vi "pmu_Read CFG3.vi"(8 "error in (no error)":errorcluster, 11 "system info in":refnum<class "PMU System Info.lvclass">) -> (0 "error out":errorcluster, 2 "CFG-3":T1={"station name"="", "PMU ID"=0, "global PMU ID"=10000000, "time base"=1, "nominal frequency"=enum."60 Hz", "reporting rate"=0, "phasor number"=0, "analog number"=0, "digital number"=0, "channel names"=[], "phasor scale first 4 bytes"=[], "phasor scale factors"=[], "phasor angle offsets [rad]"=[], "analog scale factors"=[], "analog magnitude offsets"=[], "digital units"=[], "data format"=15, "number of PMUs"=1} {"digital units" format="%.0x"}, 3 "system info out":refnum<class "PMU System Info.lvclass">)   [LabVIEW 2013, in "NI_EP_PMU.lvlib" / "PMU System Info.lvclass"]
uses:
  <vilib>/addons/Electrical Power/PMU/Common/Classes/PMU System Info/PMU System Info.lvclass
  <vilib>/addons/Electrical Power/PMU/Common/Controls/pmu_CFG-3 Class.ctl
  <vilib>/addons/Electrical Power/PMU/Common/Classes/PMU System Info/PMU System Info.lvclass/PMU System Info.ctl
  <vilib>/addons/Electrical Power/PMU/NI_EP_PMU.lvlib
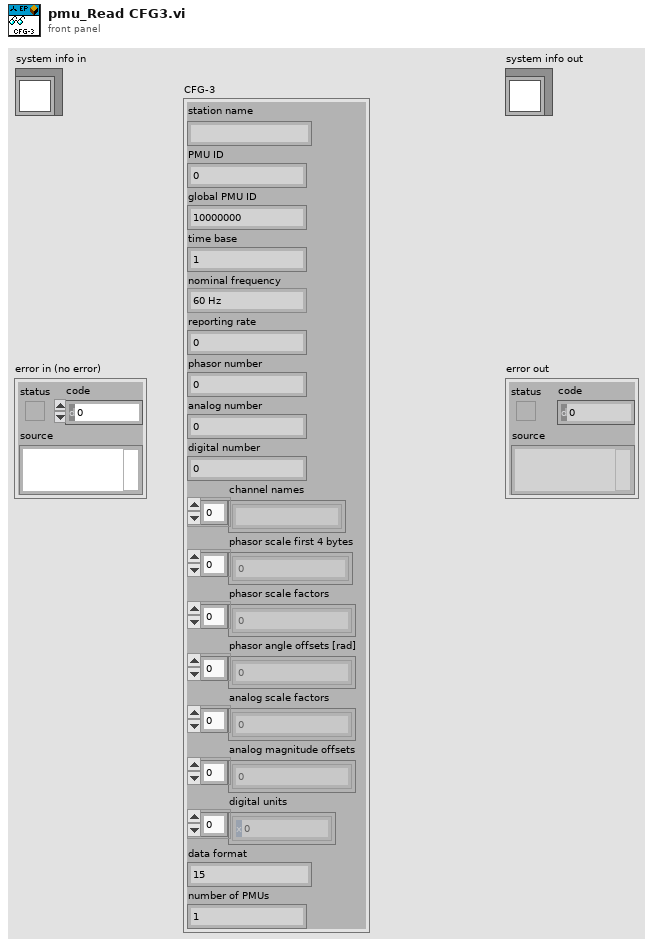
[diagram p1: front panel]
types:
  T1 = typedef "NI_EP_PMU.lvlib/pmu_CFG-3 Class.ctl" = cluster{"station name":string, "PMU ID":u16, "global PMU ID":u64, "time base":u32, "nominal frequency":enum16{"50 Hz", "60 Hz"}, "reporting rate":i16, "phasor number":u16, "analog number":u16, "digital number":u16, "channel names":string[], "phasor scale first 4 bytes":u32[], "phasor scale factors":sgl[], "phasor angle offsets [rad]":sgl[], "analog scale factors":sgl[], "analog magnitude offsets":sgl[], "digital units":u32[], "data format":u16, "number of PMUs":u16}
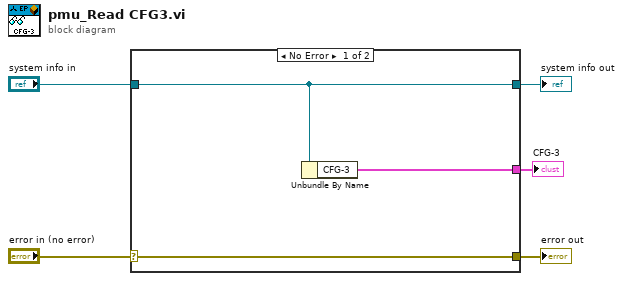
[diagram p0: block diagram]
diagram:
  n1 = case shown="No Error" "error in (no error)" {
    selector: "error in (no error)" -> [w8 w9]
    tunnel: [w8 w9] -> w4
    tunnel: [w7 w10] -> w2
    tunnel: "system info in" -> [w7 w10]
    tunnel: [w6 _] -> w1
    frame No Error {
      n2 = Unbundle By Name(w7) -> ("CFG-3"=w6:T1)
    }
    frame Error {
    }
  }
  "error out" <- w4
  "system info out" <- w2
  "CFG-3" <- w1
